vi "subfft.vi"(2 "y-signal":dbl[](array[numeric]) format="%.2f", 3 "time step":dbl format="%.2f") -> (0 "Phase":cluster{"f0":dbl, "df":dbl, "real part":dbl[]} {"real part" format="%.2f"; "df" format="%.2f"; "f0" format="%.2f"}, 1 "Amplitude":cluster{"f0":dbl, "df":dbl, "real part":dbl[]} {"real part" format="%.2f"; "df" format="%.2f"; "f0" format="%.2f"})   [LabVIEW 2010]
uses:
  <vilib>/measure/maspectr.llb/FFT Spectrum (Mag-Phase) for 1 Chan.vi
  <vilib>/measure/NI_MAPro.lvlib
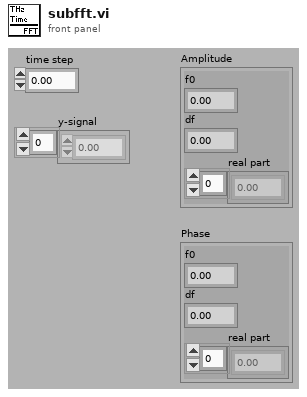
[diagram p1: front panel]
types:
  T1 = enum16{"None ", "Hanning", "Hamming", "Blackman-Harris", "Exact Blackman", "Blackman", "Flat Top", "4 Term B-Harris ", "7 Term B-Harris", "Low Sidelobe"}
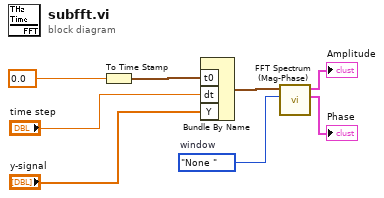
[diagram p0: block diagram]
diagram:
  w2 = T1."None "  # window
  n1 = To Time Stamp(1:0.0 ("t0")) -> (0:w1:timestamp)
  n2 = Bundle By Name("t0"=w1, "dt"="time step", "Y"="y-signal") -> (w5:waveform(dbl))  [unwired: 1 in]
  n3 = call-poly <vilib>:"FFT Spectrum (Mag-Phase).vi"("window"=w2, "time signal"=w5) -> ("phase"=→"Phase":cluster{"f0":dbl, "df":dbl, "phase":dbl[]}, "magnitude"=→"Amplitude":cluster{"f0":dbl, "df":dbl, "magnitude":dbl[]})  [unwired: 5 in, 3 out]
